vi "FLOW-BUS RW.vi"(0 "VISA resource name":refnum<visa-resource-name>, 7 "FLOW-BUS Command Settings":T1={"Node Address (3)"=3, "Communication Command"=enum."Send parameter with destination address", "Process (0)"=0, "Parameter (0)"=0, "Data Type (0: Character)"=enum."Integer", "Data for Char or Int (0)"=0, "Data for Float or Long (0)"=0.0, "Data for String"="", "Length of Requested String (0)"=0} {"Data Type (0: Character)" format="%0d"; "Communication Command" format="%0d"; "Node Address (3)" min=3 max=128}, 11 "error in (no error)":errorcluster {"code" format="%x"}) -> (4 "VISA resource name out":refnum<visa-resource-name>, 6 "Requested Char, Int or Long":u32, 8 "Requested Float or Long":sgl, 10 "Requested String":string, 15 "error out":errorcluster {"code" format="%x"})   [LabVIEW 2024, in "Bronkhorst FLOW-BUS.lvlib"]
doc: "This VI is the core of allmost all Bronkhorst FLOW-BUS Driver VI's. It is used to send FLOW-BUS commands to the selected instrument, and to decode the instruments response to those commands. Usages of this VI is as follows:\n\n - Wire up the VISA connections to their respective controls or constants.\n - To request a parameter (read), enter the values for the Node Address, Process, Parameter, and Data Type, and set the Communication Command to \"Request Parameter\"\n - To send a parameter (write), enter the values for the Node Address, Process, Parameter, Data Type, and the Data you want to send (in the Char/Int, Float/Long or String control) and set the Communication Command to \"Send paramter with destination address and 00 response\"\n- Now Run the VI"
uses:
  Bronkhorst FLOW-BUS.lvlib
  FLOW-BUS RW.ctl
panel:
  out "Formatted Command":string
  out "Received Response":string
  # "The process, parameter, and  data type values can be found in the parameter properties table on page 38 of document 9.17.027."
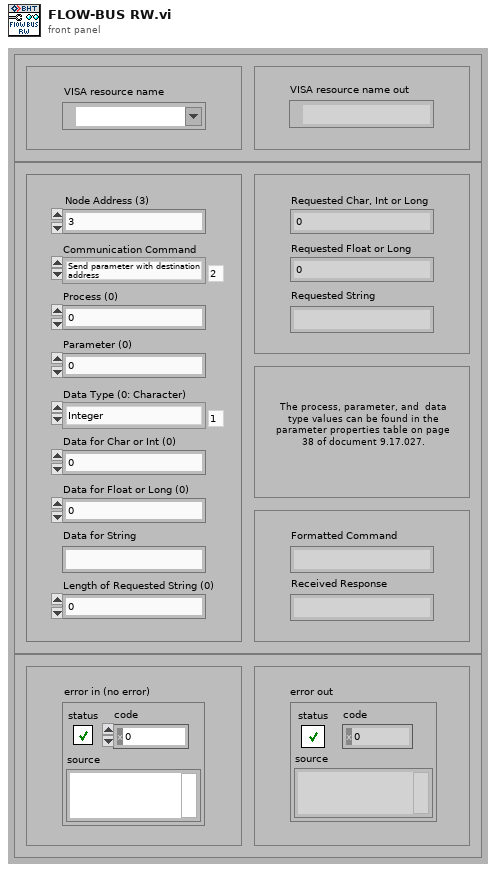
[diagram p1: front panel]
types:
  T1 = typedef "Bronkhorst FLOW-BUS.lvlib/FLOW-BUS RW.ctl" = cluster{"Node Address (3)":u8, "Communication Command":enum16{"Status message", "Send parameter with destination address and 00 response", "Send parameter with destination address", "Request parameter"}, "Process (0)":u16, "Parameter (0)":u16, "Data Type (0: Character)":enum16{"Character", "Integer", "Float or Long", "String"}, "Data for Char or Int (0)":u32, "Data for Float or Long (0)":sgl, "Data for String":string, "Length of Requested String (0)":u8}
  T2 = enum16{"Status message", "Send parameter with destination address and 00 response", "Send parameter with destination address", "Request parameter"}
  T3 = enum16{"Character", "Integer", "Float or Long", "String"}
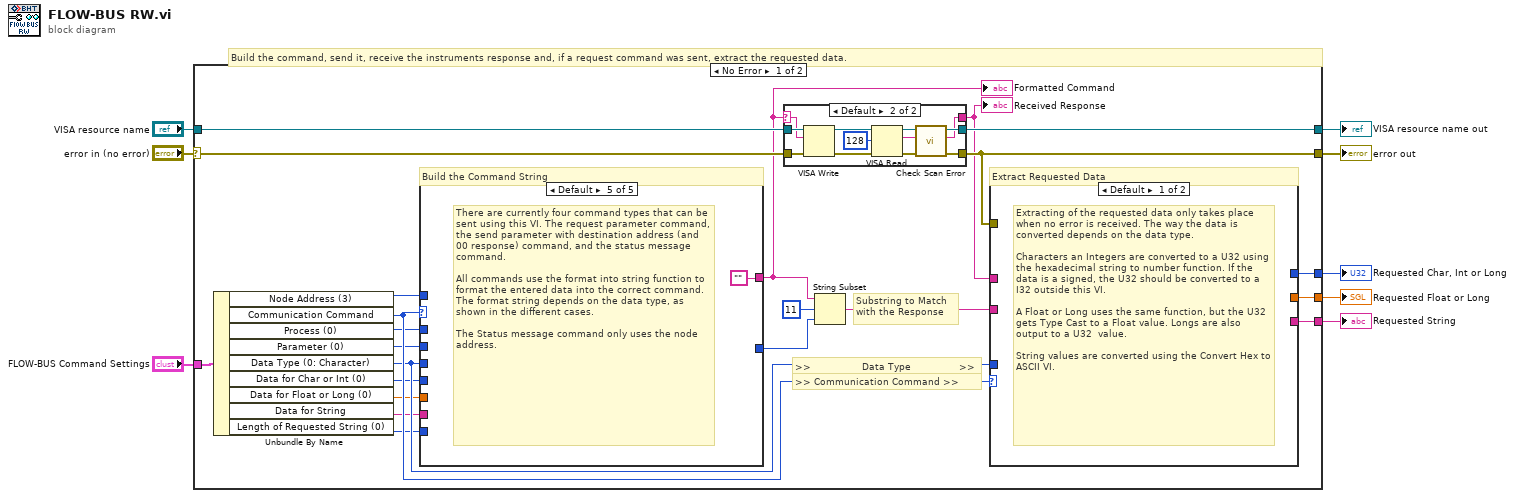
[diagram p0: block diagram]
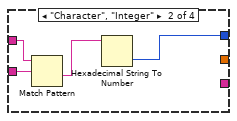
[diagram p5: hidden frame]
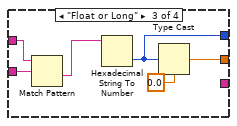
[diagram p6: hidden frame]
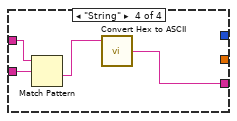
[diagram p7: hidden frame]
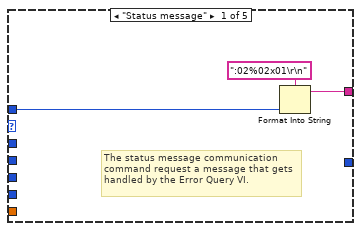
[diagram p8: hidden frame]
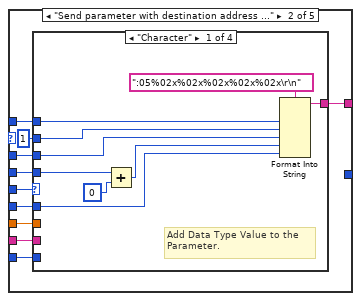
[diagram p9: hidden frame]
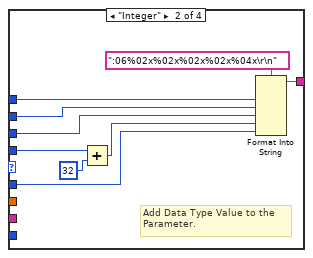
[diagram p10: hidden frame]
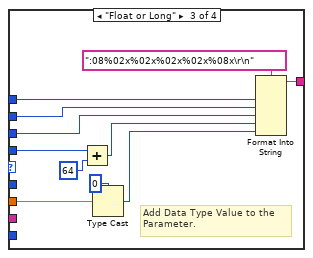
[diagram p11: hidden frame]
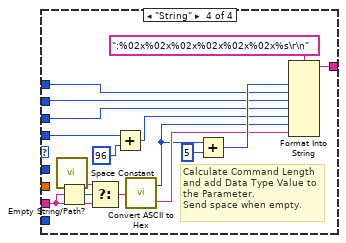
[diagram p12: hidden frame]
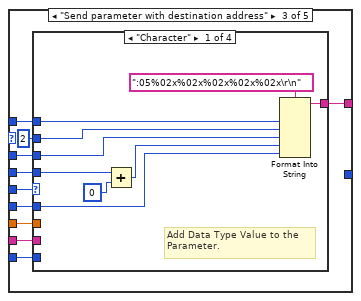
[diagram p13: hidden frame]
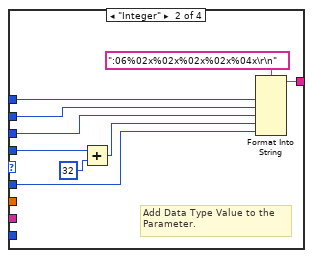
[diagram p14: hidden frame]
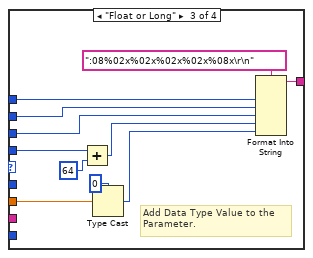
[diagram p15: hidden frame]
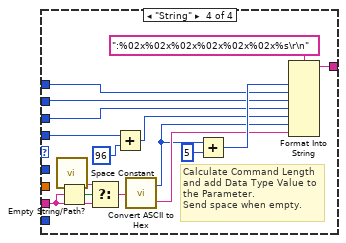
[diagram p16: hidden frame]
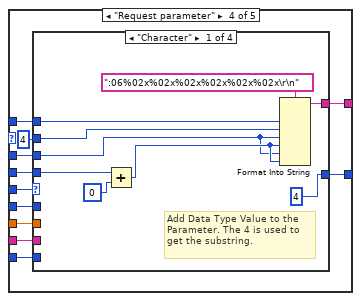
[diagram p17: hidden frame]
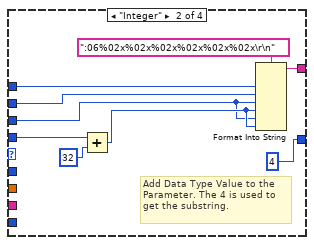
[diagram p18: hidden frame]
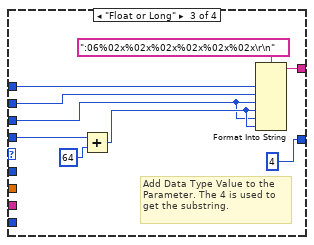
[diagram p19: hidden frame]
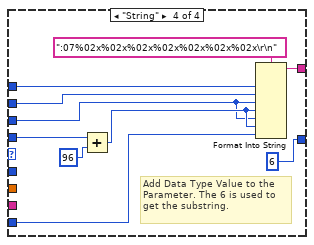
[diagram p20: hidden frame]
diagram:
  # "Build the command, send it, receive the instruments response and, if a request command was sent, extract the requested data."
  n1 = case shown="No Error" "error in (no error)" {
    selector: "error in (no error)" -> [w24 w235]
    tunnel: [w13 _] -> w8
    tunnel: [w12 w235] -> w7
    tunnel: [w15 _] -> w6
    tunnel: [w14 _] -> w5
    tunnel: [w28 w236] -> w4
    tunnel: "VISA resource name" -> [w23 w236]
    tunnel: "FLOW-BUS Command Settings" -> [w22 _]
    frame No Error {
      # "Extract Requested Data"
      # "Substring to Match\nwith the Response"
      # ">> Communication Command >>"
      # ">>                 Data Type                >>"
      # "Build the Command String"
      n2 = Unbundle By Name(w22) -> ("Node Address (3)"=w27:u8, "Communication Command"=w30:T2, "Process (0)"=w26:u16, "Parameter (0)"=w25:u16, "Data Type (0: Character)"=w29:T3, "Data for Char or Int (0)"=w21:u32, "Data for Float or Long (0)"=w20:sgl, "Data for String"=w19:string, "Length of Requested String (0)"=w18:u8)
      n3 = case shown="Default" w30 {
        tunnel: w27 -> [w74 w80 w135 w191 _]
        tunnel: w26 -> [_ w81 w136 w192 _]
        tunnel: w25 -> [_ w82 w137 w193 _]
        tunnel: w29 -> [_ w85 w140 w196 _]
        tunnel: w21 -> [_ w83 w138 w194 _]
        tunnel: w20 -> [_ w84 w139 w195 _]
        tunnel: [w73 w79 w134 w190 ""] -> w9
        tunnel: w19 -> [_ w77 w132 w189 _]
        tunnel: w18 -> [_ w78 w133 w188 _]
        tunnel: [_ _ _ w187 _] -> w16
        frame "Status message" {
          # "The status message communication command request a message that gets handled by the Error Query VI."
          n4 = Format Into String(format string=":02%02x01\r\n", w74) -> (resulting string=w73:string)  [unwired: 2 in, 1 out]
        }
        frame "Send parameter with destination address and 00 response" {
          n5 = case shown="\"Character\"" w85 {
            tunnel: w84 -> [_ _ w105 _]
            tunnel: w83 -> [w87 w95 _ _]
            tunnel: w82 -> [w90 w98 w109 w127]
            tunnel: w81 -> [w91 w99 w110 w123]
            tunnel: u8 1 -> [w86 w100 w111 w124]
            tunnel: w80 -> [w92 w101 w112 w125]
            tunnel: [w89 w97 w108 w126] -> w79
            tunnel: w78 -> [_ _ _ _]
            tunnel: w77 -> [_ _ _ w117]
            frame "Character" {
              # "Add Data Type Value to the Parameter."
              n6 = Add(x=w90, y=u16 0 ("Parameter")) -> (x+y=w93:u16)
              n7 = Format Into String(format string=":05%02x%02x%02x%02x%02x\r\n", w92, w86, w91, w93, w87) -> (resulting string=w89:string)  [unwired: 2 in, 1 out]
            }
            frame "Integer" {
              # "Add Data Type Value to the Parameter."
              n8 = Add(x=w98, y=u16 32 ("Parameter")) -> (x+y=w102:u16)
              n9 = Format Into String(format string=":06%02x%02x%02x%02x%04x\r\n", w101, w100, w99, w102, w95) -> (resulting string=w97:string)  [unwired: 2 in, 1 out]
            }
            frame "Float or Long" {
              # "Add Data Type Value to the Parameter."
              n10 = Add(x=w109, y=u16 64 ("Parameter")) -> (x+y=w113:u16)
              n11 = Type Cast(type=0, x=w105) -> (*(type *) &x=w106:i32)
              n12 = Format Into String(format string=":08%02x%02x%02x%02x%08x\r\n", w112, w111, w110, w113, w106) -> (resulting string=w108:string)  [unwired: 2 in, 1 out]
            }
            frame "String" {
              # "Calculate Command Length and add Data Type Value to the Parameter.\nSend space when empty."
              n13 = call <vilib>:"Space Constant.vi"() -> ("String"=w115:string)
              n14 = Empty String/Path?(string/path=w117) -> (empty?=w118:bool)
              n15 = Select(t=w115, s=w118, f=w117) -> (s? t:f=w116:string)
              n16 = Add(x=w127, y=u16 96 ("Parameter")) -> (x+y=w122:u16)
              n17 = call "Convert ASCII to Hex.vi"("String In"=w116) -> ("Hex ASCII String Length"=w120:i32, "Hex ASCII String Out"=w121:string)
              n18 = Add(x=w120, y=5) -> (x+y=w129:i32)
              n19 = Format Into String(format string=":%02x%02x%02x%02x%02x%02x%s\r\n", w129, w125, w124, w123, w122, w120, w121) -> (resulting string=w126:string)  [unwired: 2 in, 1 out]
            }
          }
        }
        frame "Send parameter with destination address" {
          n20 = case shown="\"Character\"" w140 {
            tunnel: w139 -> [_ _ w160 _]
            tunnel: w138 -> [w142 w150 _ _]
            tunnel: w137 -> [w145 w153 w164 w182]
            tunnel: w136 -> [w146 w154 w165 w178]
            tunnel: u8 2 -> [w141 w155 w166 w179]
            tunnel: w135 -> [w147 w156 w167 w180]
            tunnel: [w144 w152 w163 w181] -> w134
            tunnel: w133 -> [_ _ _ _]
            tunnel: w132 -> [_ _ _ w171]
            frame "Character" {
              # "Add Data Type Value to the Parameter."
              n21 = Add(x=w145, y=u16 0 ("Parameter")) -> (x+y=w148:u16)
              n22 = Format Into String(format string=":05%02x%02x%02x%02x%02x\r\n", w147, w141, w146, w148, w142) -> (resulting string=w144:string)  [unwired: 2 in, 1 out]
            }
            frame "Integer" {
              # "Add Data Type Value to the Parameter."
              n23 = Add(x=w153, y=u16 32 ("Parameter")) -> (x+y=w157:u16)
              n24 = Format Into String(format string=":06%02x%02x%02x%02x%04x\r\n", w156, w155, w154, w157, w150) -> (resulting string=w152:string)  [unwired: 2 in, 1 out]
            }
            frame "Float or Long" {
              # "Add Data Type Value to the Parameter."
              n25 = Add(x=w164, y=u16 64 ("Parameter")) -> (x+y=w168:u16)
              n26 = Type Cast(type=0, x=w160) -> (*(type *) &x=w161:i32)
              n27 = Format Into String(format string=":08%02x%02x%02x%02x%08x\r\n", w167, w166, w165, w168, w161) -> (resulting string=w163:string)  [unwired: 2 in, 1 out]
            }
            frame "String" {
              # "Calculate Command Length and add Data Type Value to the Parameter.\nSend space when empty."
              n28 = call <vilib>:"Space Constant.vi"() -> ("String"=w172:string)
              n29 = Empty String/Path?(string/path=w171) -> (empty?=w173:bool)
              n30 = Select(t=w172, s=w173, f=w171) -> (s? t:f=w170:string)
              n31 = Add(x=w182, y=u16 96 ("Parameter")) -> (x+y=w177:u16)
              n32 = call "Convert ASCII to Hex.vi"("String In"=w170) -> ("Hex ASCII String Length"=w175:i32, "Hex ASCII String Out"=w176:string)
              n33 = Add(x=w175, y=5) -> (x+y=w184:i32)
              n34 = Format Into String(format string=":%02x%02x%02x%02x%02x%02x%s\r\n", w184, w180, w179, w178, w177, w175, w176) -> (resulting string=w181:string)  [unwired: 2 in, 1 out]
            }
          }
        }
        frame "Request parameter" {
          n35 = case shown="\"Character\"" w196 {
            tunnel: w195 -> [_ _ _ _]
            tunnel: w194 -> [_ _ _ _]
            tunnel: w193 -> [w204 w213 w222 w232]
            tunnel: w192 -> [w203 w212 w221 w231]
            tunnel: u8 4 -> [w202 w211 w220 w230]
            tunnel: w191 -> [w201 w210 w219 w229]
            tunnel: [w199 w208 w217 w227] -> w190
            tunnel: w189 -> [_ _ _ _]
            tunnel: w188 -> [_ _ _ w226]
            tunnel: [4 ("offset (0)") 4 ("offset (0)") 4 ("offset (0)") 6 ("offset (0)")] -> w187
            frame "Character" {
              # "Add Data Type Value to the Parameter. The 4 is used to get the substring."
              n36 = Add(x=w204, y=u16 0 ("Parameter")) -> (x+y=w205:u16)
              n37 = Format Into String(format string=":06%02x%02x%02x%02x%02x%02x\r\n", w201, w202, w203, w205, w203, w205) -> (resulting string=w199:string)  [unwired: 2 in, 1 out]
            }
            frame "Integer" {
              # "Add Data Type Value to the Parameter. The 4 is used to get the substring."
              n38 = Add(x=w213, y=u16 32 ("Parameter")) -> (x+y=w214:u16)
              n39 = Format Into String(format string=":06%02x%02x%02x%02x%02x%02x\r\n", w210, w211, w212, w214, w212, w214) -> (resulting string=w208:string)  [unwired: 2 in, 1 out]
            }
            frame "Float or Long" {
              # "Add Data Type Value to the Parameter. The 4 is used to get the substring."
              n40 = Add(x=w222, y=u16 64 ("Parameter")) -> (x+y=w223:u16)
              n41 = Format Into String(format string=":06%02x%02x%02x%02x%02x%02x\r\n", w219, w220, w221, w223, w221, w223) -> (resulting string=w217:string)  [unwired: 2 in, 1 out]
            }
            frame "String" {
              # "Add Data Type Value to the Parameter. The 6 is used to get the substring."
              n42 = Add(x=w232, y=u16 96 ("Parameter")) -> (x+y=w233:u16)
              n43 = Format Into String(format string=":07%02x%02x%02x%02x%02x%02x%02x\r\n", w229, w230, w231, w233, w231, w233, w226) -> (resulting string=w227:string)  [unwired: 2 in, 1 out]
            }
          }
        }
        frame Default {
          # "There are currently four command types that can be sent using this VI. The request parameter command, the send parameter with destination address (and 00 response) command, and the status message command.\n \nAll commands use the format into string function to format the entered data into the correct command. The format string depends on the data type, as shown in the different cases. \n\nThe Status message command only uses the node address."
        }
      }
      "Formatted Command" <- w9
      n44 = case shown="Default" w9 {
        selector: w9 -> [w31 w34]
        tunnel: [w33 w39] -> w28
        tunnel: w24 -> [w32 w38]
        tunnel: w23 -> [w33 w37]
        tunnel: [w32 w36] -> w12
        tunnel: [w31 w35] -> w10
        frame "" {
          # "Unsupported Command"
        }
        frame Default {
          n45 = VISA Write(VISA resource name=w37, write buffer=w34, error in (no error)=w38) -> (VISA resource name out=w40:refnum<visa-resource-name>, error out=w41:errorcluster)  [unwired: 1 out]
          n46 = VISA Read(VISA resource name=w40, byte count=u32 128, error in (no error)=w41) -> (VISA resource name out=w43:refnum<visa-resource-name>, read buffer=w44:string, error out=w45:errorcluster)  [unwired: 1 out]
          n47 = call "Check Scan Error.vi"("error in (no error)"=w45, "Response Input"=w44, "VISA resource name"=w43) -> ("error out"=w36:errorcluster, "Response Output"=w35:string, "VISA resource name out"=w39:refnum<visa-resource-name>)  [unwired: 6 in]
        }
      }
      "Received Response" <- w10
      n48 = String Subset(string=w9, offset (0)=11, length (rest)=w16) -> (substring=w11:string)
      n49 = case shown="Default" w30 {
        tunnel: [_ w48] -> w15
        tunnel: [_ w47] -> w14
        tunnel: [_ w46] -> w13
        tunnel: w12 -> [_ w49]
        tunnel: w10 -> [_ w52]
        tunnel: w11 -> [_ w51]
        tunnel: w29 -> [_ w50]
        frame Default {
          # "Extracting of the requested data only takes place when no error is received. The way the data is converted depends on the data type. \n\nCharacters an Integers are converted to a U32 using the hexadecimal string to number function. If the data is a signed, the U32 should be converted to a I32 outside this VI.\n\nA Float or Long uses the same function, but the U32 gets Type Cast to a Float value. Longs are also output to a U32  value.\n\nString values are converted using the Convert Hex to ASCII VI."
        }
        frame "Request parameter" {
          n50 = case shown="No Error" w49 {
            tunnel: [_ w58] -> w48
            tunnel: [_ w57] -> w47
            tunnel: [_ w56] -> w46
            tunnel: w52 -> [_ w55]
            tunnel: w50 -> [_ w54]
            tunnel: w51 -> [_ w53]
            frame Error {
            }
            frame No Error {
              n51 = case shown="Default" w54 {
                tunnel: w55 -> [_ w60 w65 w69]
                tunnel: [_ _ w67 _] -> w57
                tunnel: [_ _ _ w72] -> w58
                tunnel: [_ w62 w66 _] -> w56
                tunnel: w53 -> [_ w61 w64 w71]
                frame Default {
                  # "The substring is used to select where in the response the data is located. \n\nIf this is not used, and corrupt data is received and read from a fixed position, false values will be displayed in the indicators."
                }
                frame "Character", "Integer" {
                  n52 = Match Pattern(string=w60, regular expression=w61) -> (after substring=w59:string)  [unwired: 1 in, 3 out]
                  n53 = Hexadecimal String To Number(string=w59) -> (number=w62:u32)  [unwired: 2 in, 1 out]
                }
                frame "Float or Long" {
                  n54 = Match Pattern(string=w65, regular expression=w64) -> (after substring=w63:string)  [unwired: 1 in, 3 out]
                  n55 = Hexadecimal String To Number(string=w63) -> (number=w66:u32)  [unwired: 2 in, 1 out]
                  n56 = Type Cast(type=sgl 0.0, x=w66) -> (*(type *) &x=w67:sgl)
                }
                frame "String" {
                  n57 = Match Pattern(string=w69, regular expression=w71) -> (after substring=w70:string)  [unwired: 1 in, 3 out]
                  n58 = call "Convert Hex to ASCII.vi"("Hex String"=w70) -> ("ASCII String"=w72:string)  [unwired: 1 in]
                }
              }
            }
          }
        }
      }
    }
    frame Error {
    }
  }
  "VISA resource name out" <- w4
  "error out" <- w7
  "Requested Float or Long" <- w5
  "Requested String" <- w6
  "Requested Char, Int or Long" <- w8
